vi "BRig_Host__Loop_Consumer_RunState__getThresholds__getData.vi"(10 "input_idx":i32[](array[numeric]), 11 "input_dataTS":u16[][](array[numeric])) -> (3 "output_data":u16[](array[numeric]))   [LabVIEW 2014]
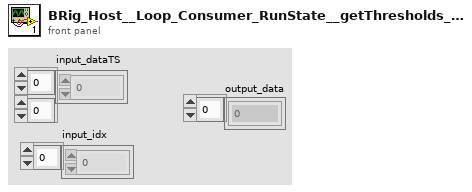
[diagram p1: front panel]
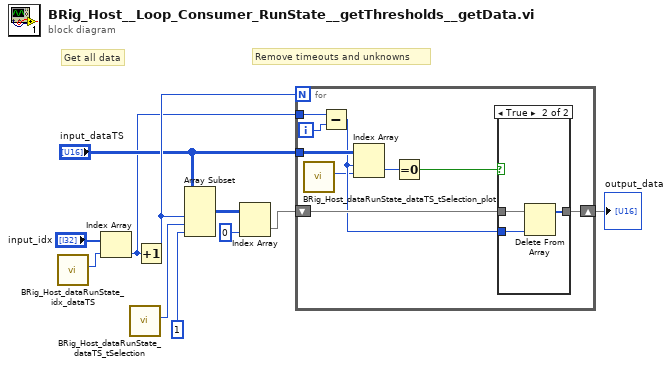
[diagram p0: block diagram]
diagram:
  # "Remove timeouts and unknowns"
  # "Get all data"
  n1 = call "BRig_Host_dataRunState_idx_dataTS.vi"() -> ("output_idx_dataTS"=w10:i32)  [unwired: 11 in]
  n2 = Index Array(array="input_idx", index=w10) -> (element=w5:i32)
  n3 = call "BRig_Host_dataRunState_dataTS_tSelection.vi"() -> ("output_idx_dataTS_tSelection"=w9:i32)  [unwired: 11 in]
  n4 = Increment(x=w5) -> (x+1=w7:i32)
  n5 = Array Subset(array="input_dataTS", length (row)=w7, index (col)=w9, length (col)=1 ("length")) -> (w4:u16[][])  [unwired: 1 in]
  n6 = Index Array(array=w4, index (col)=0 ("disabled index (col)")) -> (element=w2:u16[])  [unwired: 1 in]
  n7 = for {
    N: w7 -> [_]
    shift-right: [w14] -> w1
    shift-left: w2 -> [w17]
    tunnel: "input_dataTS" -> [w20]
    tunnel: w5 -> [w16]
    i -> [w19]
    n8 = call "BRig_Host_dataRunState_dataTS_tSelection_plot.vi"() -> ("output_idx_dataTS_tSelection_plot"=w13:i32)  [unwired: 11 in]
    n9 = Subtract(x=w16, y=w19) -> (x-y=w15:i32)
    n10 = Index Array(array=w20, index (row)=w15, index (col)=w13) -> (element=w18:u16)
    n11 = Equal To 0?(x=w18) -> (x = 0?=w12:bool)
    n12 = case shown="True" w12 {
      tunnel: w17 -> [w21 w24]
      tunnel: w15 -> [_ w23]
      tunnel: [w21 w22] -> w14
      frame False {
      }
      frame True {
        n13 = Delete From Array(array=w24, index=w23) -> (array with subset deleted=w22:u16[])  [unwired: 1 in, 1 out]
      }
    }
  }
  "output_data" <- w1
